vi "RT FIFO Initialize.vi"(11 "name (unnamed)":string) -> (0 "Queue Error":errorcluster, 3 "rt fifo":refnum<k33>)   [LabVIEW 2020]
panel:
  out "Queue Error 2":errorcluster
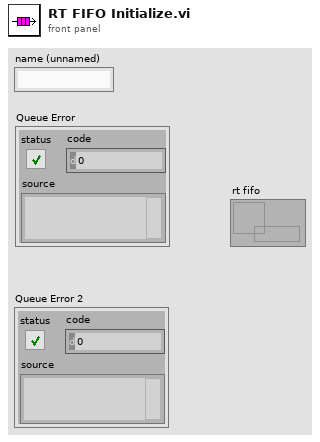
[diagram p1: front panel]
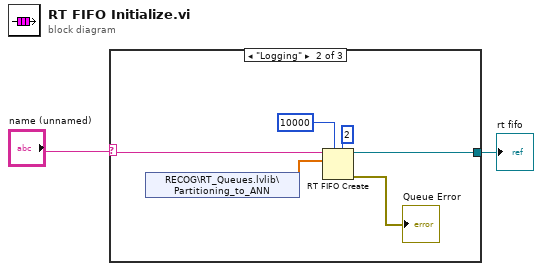
[diagram p0: block diagram]
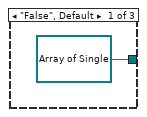
[diagram p2: hidden frame]
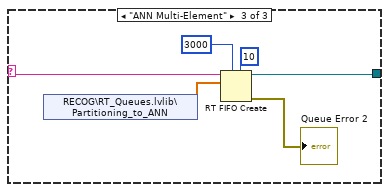
[diagram p3: hidden frame]
diagram:
  n1 = case shown="\"Logging\"" "name (unnamed)" {
    selector: "name (unnamed)" -> [_ w9 w11]
    tunnel: [refnum<k33> refnum ("rt fifo") w4 w10] -> w1
    frame "False", Default {
    }
    frame "Logging" {
      n2 = shared-variable "RECOG\\RT_Queues.lvlib\\Partitioning_to_ANN"() -> (w5:sgl[])  [unwired: 1 in, 1 out]
      n3 = RT FIFO Create(0:w9, 1:w5, 4:u32 10000 ("size (10)"), 6:u32 2 ("elements in array (1)")) -> (8:w4:refnum<k33>, 11:→"Queue Error":errorcluster)  [unwired: 4 in, 1 out]
    }
    frame "ANN Multi-Element" {
      n4 = shared-variable "RECOG\\RT_Queues.lvlib\\Partitioning_to_ANN"() -> (w12:sgl[])  [unwired: 1 in, 1 out]
      n5 = RT FIFO Create(0:w11, 1:w12, 4:u32 3000 ("size (10)"), 6:u32 10 ("elements in array (1)")) -> (8:w10:refnum<k33>, 11:→"Queue Error 2":errorcluster)  [unwired: 4 in, 1 out]
    }
  }
  "rt fifo" <- w1
